vi "Turn Right.vi"   [LabVIEW 2019]
uses:
  Robot Global Data.vi
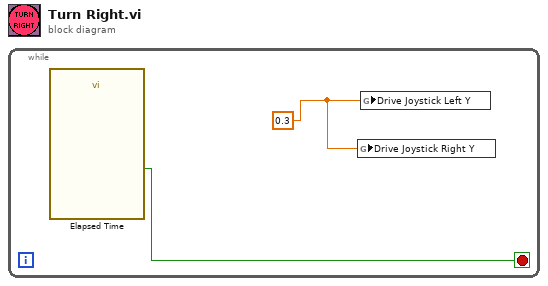
[diagram p0: block diagram]
diagram:
  n1 = while {
    stop <- w2 stop-if-true
    w1 = 0.3
    n2 = call "Elapsed Time"() -> ("Time has Elapsed"=w2:bool)  [unwired: 12 in, 7 out]
    n3 = global write "Robot Global Data.vi" "Drive Joystick Right Y"(w1) -> ()
    n4 = global write "Robot Global Data.vi" "Drive Joystick Left Y"(w1) -> ()
  }
